vi "ArthOps.vi"() -> ()   [LabVIEW 2024]
panel:
  out "x*2^n":dbl
  in  "x":dbl
  in  "y":dbl
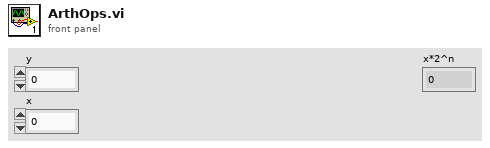
[diagram p1: front panel]
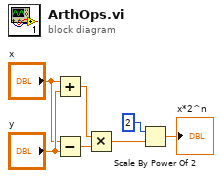
[diagram p0: block diagram]
diagram:
  n1 = Add(x="x", y="y") -> (x+y=w5:dbl)
  n2 = Subtract(x="x", y="y") -> (x-y=w4:dbl)
  n3 = Multiply(x=w5, y=w4) -> (x*y=w3:dbl)
  n4 = Scale By Power Of 2(n=i16 2, x=w3) -> (x*2^n=→"x*2^n":dbl)
